vi "niFPGA BW CU Order 2 (32-bit).vi"(0 "filter state in":T1, 1 "reset":bool, 5 "input data":i32, 7 "accumulator in":fxp<+/-,36,32>, 9 "adder in":fxp<+/-,34,34>, 11 "iteration":u8, 12 "in shift":i8=-1, 13 "lowpass?":bool) -> (4 "filter state out":T1, 6 "state to multiply":i32, 8 "accumulator out":fxp<+/-,36,32> format="%.14g", 10 "adder out":fxp<+/-,34,34>, 15 "terminate":bool)   [LabVIEW 2017]
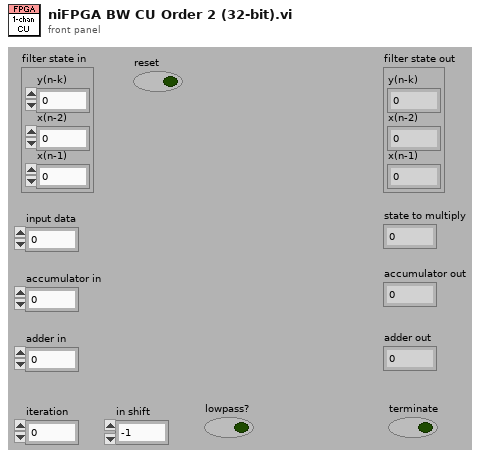
[diagram p1: front panel]
types:
  T1 = cluster{"y(n-k)":i32, "x(n-2)":i32, "x(n-1)":i32}
  T2 = cluster{"y(n-1)":i32, "x(n-2)":i32, "x(n-1)":i32}
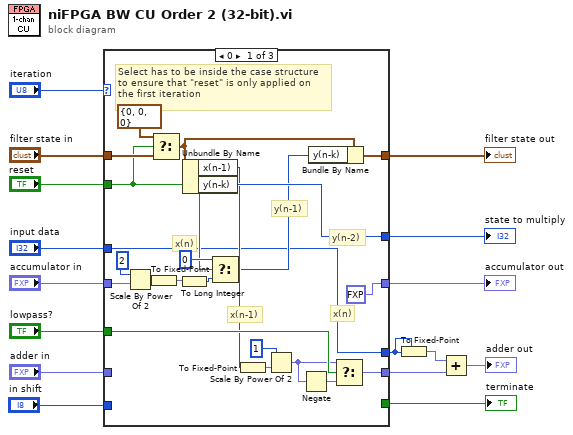
[diagram p0: block diagram]
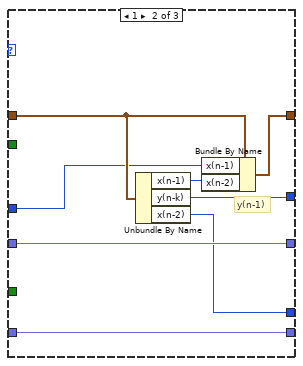
[diagram p2: hidden frame]
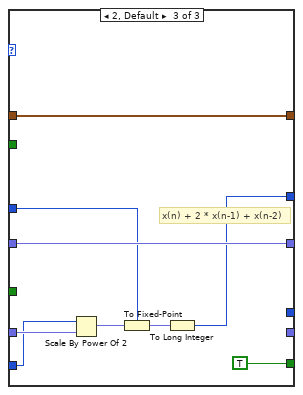
[diagram p3: hidden frame]
diagram:
  n1 = case shown="0" "iteration" {
    tunnel: [w38 w40 w54] -> w11
    tunnel: "input data" -> [w23 w39 w48]
    tunnel: [w27 w46 _] -> w6
    tunnel: "adder in" -> [_ w46 w53]
    tunnel: [w36 w45 w49] -> w10
    tunnel: [w23 w43 _] -> w5
    tunnel: [fxp<+/-,36,32> 0.0 ("Numeric") w44 w51] -> w9
    tunnel: [_ _ TRUE] -> w8
    tunnel: "reset" -> [w31 _ _]
    tunnel: "accumulator in" -> [w21 w44 w51]
    tunnel: "filter state in" -> [w32 w41 w54]
    tunnel: "lowpass?" -> [w29 _ _]
    tunnel: "in shift" -> [_ _ w47]
    frame 0 {
      # "y(n-1)"
      # "Select has to be inside the case structure\nto ensure that \"reset\" is only applied on\nthe first iteration"
      # "x(n)"
      # "x(n)"
      # "x(n-1)"
      # "y(n-2)"
      n2 = Scale By Power Of 2(n=2, x=w21) -> (x*2^n=w19:fxp<+/-,36,32>)
      n3 = To Fixed-Point(number=w19) -> (fixed-point=w22:fxp<+/-,32,32>)  [unwired: 1 out]
      n4 = Select(t=T2 {"y(n-1)"=0, "x(n-2)"=0, "x(n-1)"=0} ("output cluster"), s=w31, f=w32) -> (s? t:f=w34:T1)
      n5 = To Long Integer(number=w22) -> (32bit integer=w18:i32)
      n6 = Unbundle By Name(w34) -> ("x(n-1)"=w26:i32, "y(n-k)"=w36:i32)
      n7 = Select(t=0, s=w31, f=w18) -> (s? t:f=w24:i32)
      n8 = To Fixed-Point(number=w26) -> (fixed-point=w25:fxp<+/-,33,33>)  [unwired: 1 out]
      n9 = Scale By Power Of 2(n=1, x=w25) -> (x*2^n=w28:fxp<+/-,33,33>)
      n10 = Negate(x=w28) -> (-x=w30:fxp<+/-,34,34>)
      n11 = Bundle By Name(cluster=w34, "y(n-k)"=w24) -> (w38:T1)
      n12 = Select(t=w28, s=w29, f=w30) -> (s? t:f=w27:fxp<+/-,34,34>)
    }
    frame 1 {
      # "y(n-1)"
      n13 = Unbundle By Name(w41) -> ("x(n-1)"=w42:i32, "y(n-k)"=w45:i32, "x(n-2)"=w43:i32)
      n14 = Bundle By Name(cluster=w41, "x(n-1)"=w39, "x(n-2)"=w42) -> (w40:T1)
    }
    frame 2, Default {
      # "x(n) + 2 * x(n-1) + x(n-2)"
      n15 = Scale By Power Of 2(n=w47, x=w53) -> (x*2^n=w52:fxp<+/-,34,34>)
      n16 = To Fixed-Point(fixed-point type=w48, number=w52) -> (fixed-point=w50:fxp<+/-,32,32>)
      n17 = To Long Integer(number=w50) -> (32bit integer=w49:i32)
    }
  }
  "filter state out" <- w11
  "state to multiply" <- w10
  "terminate" <- w8
  "accumulator out" <- w9
  n18 = To Fixed-Point(fixed-point type=w5, number=w5) -> (fixed-point=w4:fxp<+/-,32,32>)
  n19 = Add(x=w4, y=w6) -> (x+y=→"adder out":fxp<+/-,34,34>)
